vi "XPARTD_StartDisp.vi"(4 "id":string, 5 "xpapath":string, 6 "force":bool, 7 "parg":string=" -p 0", 8 "error in (no error)":errorcluster, 9 "args":string, 10 "dispdev":string="${PAN_ROOT_FPAS}/_nodeID_/config/RTD/imt1i:${PAN_ROOT_FPAS}/_nodeID_/config/RTD/im1o\nfifo:${PAN_ROOT_FPAS}/_nodeID_/RTD/imt1i:${PAN_ROOT_FPAS}/_nodeID_/RTD/imt1o", 11 "iniexec":string) -> (0 "error out":errorcluster, 2 "response":string)   [LabVIEW 2016]
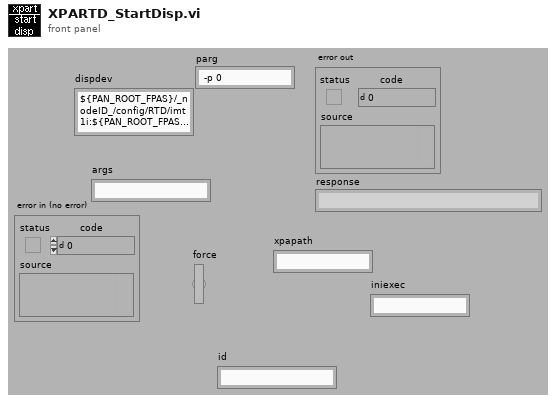
[diagram p1: front panel]
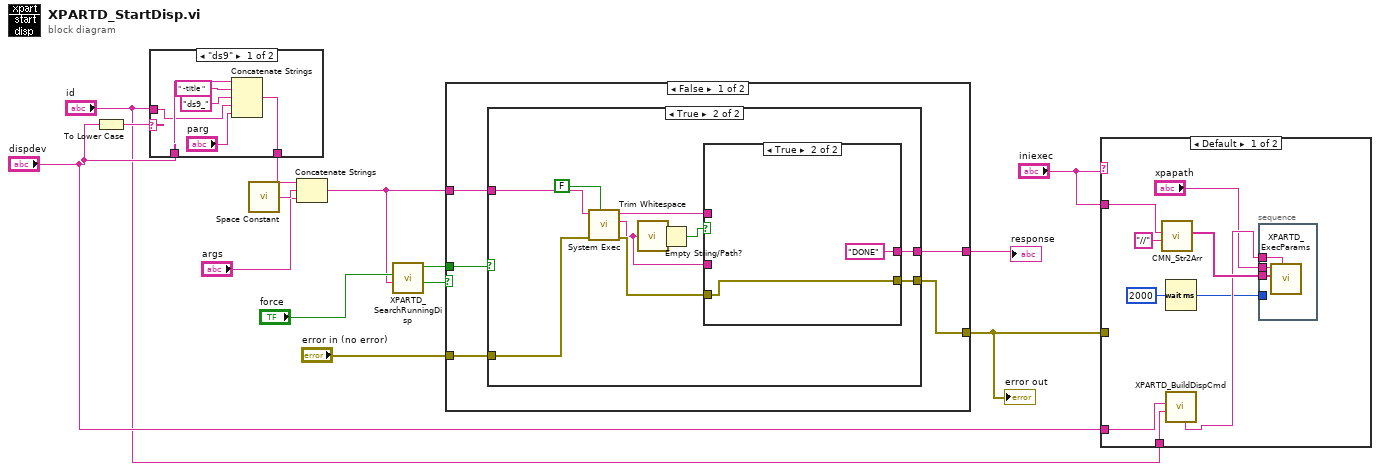
[diagram p0: block diagram]
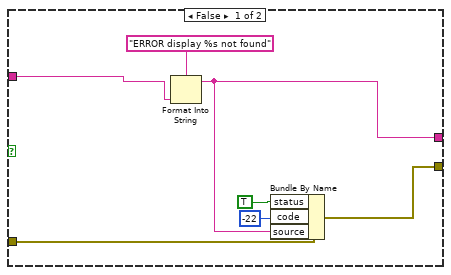
[diagram p4: hidden frame]
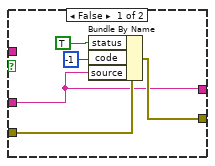
[diagram p5: hidden frame]
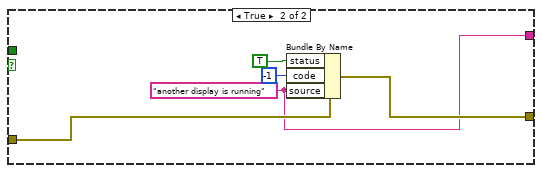
[diagram p6: hidden frame]
diagram:
  n1 = To Lower Case(string="dispdev") -> (all lower case string=w5:string)
  n2 = case shown="\"ds9\"" w5 {
    tunnel: "dispdev" -> [w20 w21]
    tunnel: [w18 w21] -> w6
    tunnel: "id" -> [w16 _]
    frame "ds9" {
      n3 = Concatenate Strings(w20, " -title " ("string"), "ds9_" ("string"), w16, "parg") -> (w18:string)
    }
    frame Default {
    }
  }
  n4 = call <vilib>:"Space Constant.vi"() -> ("String"=w14:string)
  n5 = Concatenate Strings(w6, w14, "args") -> (w11:string)
  n6 = call "XPARTD_SearchRunningDisp.vi"("display"=w11, "kill"="force") -> ("any?"=w9:bool, "exists?"=w7:bool)  [unwired: 1 in, 7 out]
  n7 = case shown="False" w9 {
    tunnel: w11 -> [w26 _]
    tunnel: "error in (no error)" -> [w25 w55]
    tunnel: [w24 w54] -> w4
    tunnel: [w23 w51] -> w8
    tunnel: w7 -> [w22 _]
    frame False {
      n8 = case shown="True" w22 {
        tunnel: w26 -> [w28 w37]
        tunnel: w25 -> [w33 w36]
        tunnel: [w32 w35] -> w24
        tunnel: [w27 w34] -> w23
        frame False {
          n9 = Format Into String(format string="ERROR display %s not found", w28) -> (resulting string=w27:string)  [unwired: 2 in, 1 out]
          n10 = Bundle By Name(cluster=w33, "status"=TRUE, "code"=-22, "source"=w27) -> (w32:errorcluster)
        }
        frame True {
          n11 = call <vilib>:"System Exec.vi"("wait until completion? (T)"=FALSE, "error in (no error)"=w36, "command line"=w37) -> ("error out"=w41:errorcluster, "standard error"=w40:string, "standard output"=w39:string)  [unwired: 3 in, 3 out]
          n12 = call <vilib>:"Trim Whitespace.vi"("string"=w40) -> ("trimmed string"=w43:string)  [unwired: 1 in]
          n13 = Empty String/Path?(string/path=w43) -> (empty?=w42:bool)
          n14 = case shown="True" w42 {
            tunnel: w41 -> [w48 w50]
            tunnel: [w47 w50] -> w35
            tunnel: w40 -> [w44 _]
            tunnel: [w44 "DONE" ("standard error")] -> w34
            tunnel: w39 -> [_ _]
            frame False {
              n15 = Bundle By Name(cluster=w48, "status"=TRUE, "code"=-1, "source"=w44) -> (w47:errorcluster)
            }
            frame True {
            }
          }
        }
      }
    }
    frame True {
      w51 = "another display is running" ("source")
      n16 = Bundle By Name(cluster=w55, "status"=TRUE, "code"=-1, "source"=w51) -> (w54:errorcluster)
    }
  }
  "error out" <- w4
  "response" <- w8
  n17 = case shown="Default" "iniexec" {
    tunnel: w4 -> [_ _]
    tunnel: "iniexec" -> [w63 _]
    tunnel: "dispdev" -> [w61 _]
    tunnel: "id" -> [w60 _]
    frame Default {
      n18 = call "CMN_Str2Arr.vi"("separator"="//", "string in"=w63) -> ("Array out"=w62:string[])  [unwired: 2 in, 7 out]
      n19 = Wait (ms)(milliseconds to wait=u32 2000) -> (millisecond timer value=w57:u32)
      n20 = call "XPARTD_BuildDispCmd.vi"("nodeID"=w60, "device in"=w61) -> ("device out"=w59:string)  [unwired: 1 in, 8 out]
      n21 = stacked-sequence {
        tunnel: w62 -> [w67]
        tunnel: w59 -> [w66]
        tunnel: "xpapath" -> [w65]
        tunnel: w57 -> [_]
        frame #0 {
          n22 = call "XPARTD_ExecParams.vi"("display"=w66, "params in"=w67, "xpapath"=w65) -> ()  [unwired: 1 in, 8 out]
        }
      }
    }
    frame "", "none" {
    }
  }
